vi "Get Plugin UI.vi"(8 "error in (no error)":errorcluster, 11 "Component UI in":refnum<class "Core Component User Interfaces.lvclass">) -> (0 "error out":errorcluster, 2 "Plugin Settings UI":refnum<class "User Interface.lvclass">, 3 "Component UI out":refnum<class "Core Component User Interfaces.lvclass">)   [LabVIEW 2017, in "DSF Core.lvlib" / "Core Component User Interfaces.lvclass"]
uses:
  Core Component User Interfaces.lvclass
  User Interface/User Interface.lvclass
  User Interface/Core/Plugin/Core Plugin User Interface.lvclass
  C:/Git/DSF/Core/Classes/User Interface/User Interface.lvclass
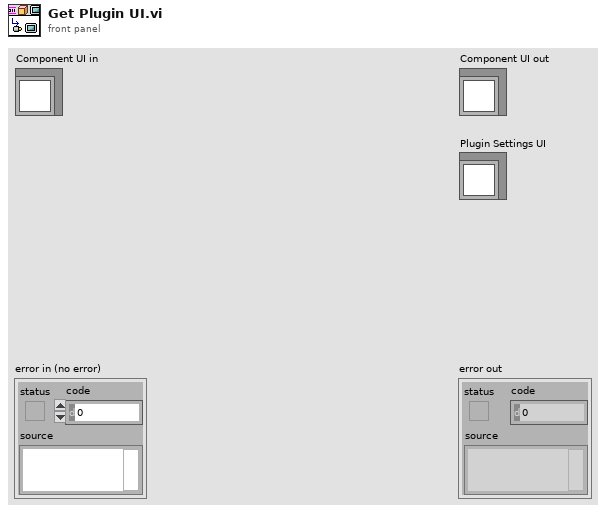
[diagram p1: front panel]
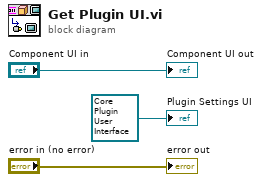
[diagram p0: block diagram]
diagram:
  "error out" <- "error in (no error)"
  "Component UI out" <- "Component UI in"
  "Plugin Settings UI" <- refnum<class "Core Plugin User Interface.lvclass"> refnum ("DSF Core.lvlib:Core Plugin User Interface.lvclass")
